vi "Write Value.vi"(8 "error in (no error)":errorcluster, 10 "Value":dbl, 11 "Sample in":refnum<class "Sample.lvclass">) -> (0 "error out":errorcluster, 3 "Sample out":refnum<class "Sample.lvclass">)   [LabVIEW 2020, in "Metrics.lvlib" / "Sample.lvclass"]
uses:
  Sample.lvclass
  Sample.lvclass/Sample.ctl
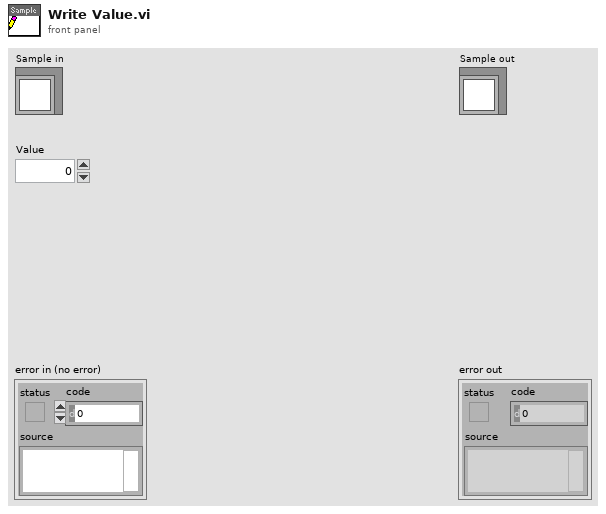
[diagram p1: front panel]
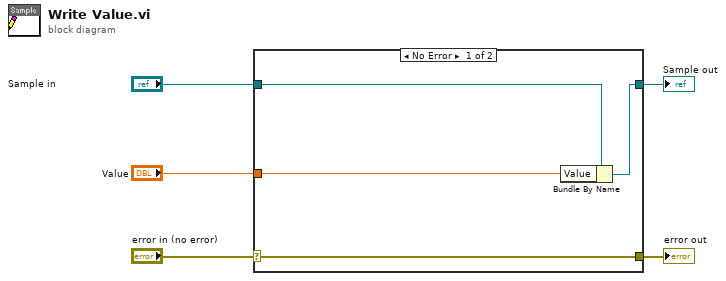
[diagram p0: block diagram]
diagram:
  n1 = case shown="No Error" "error in (no error)" {
    selector: "error in (no error)" -> [w9 w10]
    tunnel: [w9 w10] -> w4
    tunnel: [w7 w11] -> w2
    tunnel: "Sample in" -> [w8 w11]
    tunnel: "Value" -> [w6 _]
    frame No Error {
      n2 = Bundle By Name(cluster=w8, "Value"=w6) -> (w7:refnum<class "Sample.lvclass">)
    }
    frame Error {
    }
  }
  "error out" <- w4
  "Sample out" <- w2
